vi "Benchmark mupLib_parse_and_eval.vi"(8 "error in (no error)":errorcluster, 10 "Iterations":i32, 11 "Expression":string) -> (0 "error out":errorcluster, 2 "x":dbl[](array[numeric]), 3 "y":dbl[](array[numeric]), 5 "dt average":dbl)   [LabVIEW 2015]
uses:
  mupLib/mupCheckError.vi
  mupLib/mupLibPath.vi
  <vilib>/Utility/error.llb/Error Cluster From Error Code.vi
  mupLib/mupLib.lvlib
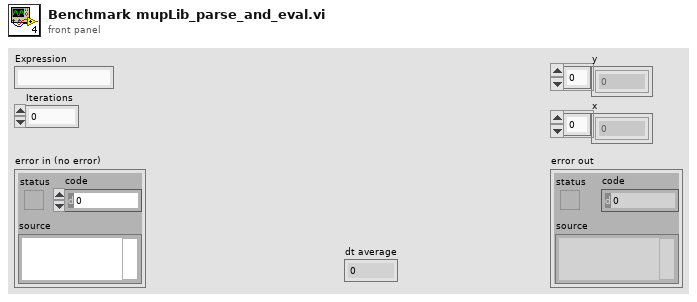
[diagram p1: front panel]
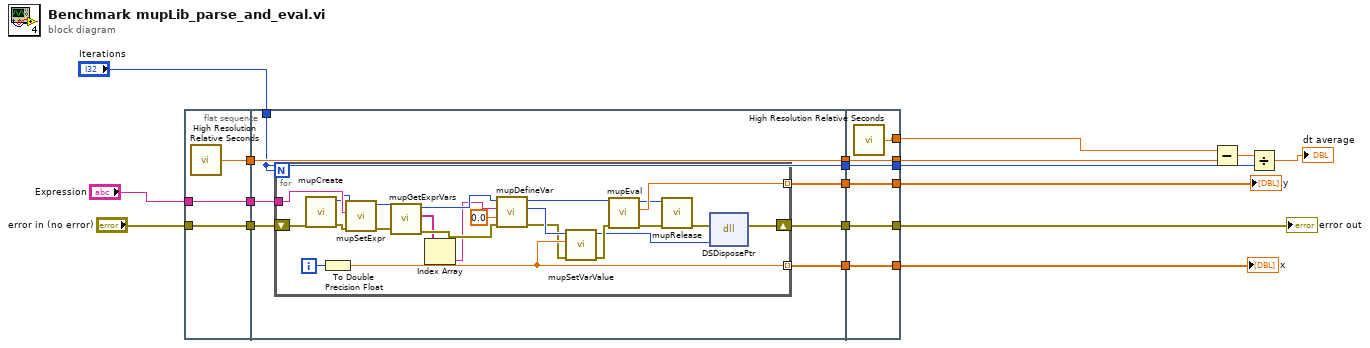
[diagram p0: block diagram]
diagram:
  n1 = flat-sequence {
    tunnel: [w22] -> w17
    tunnel: [w21] -> w12
    tunnel: [w20] -> w1
    tunnel: "error in (no error)" -> [w22]
    tunnel: "Expression" -> [w20]
    tunnel: w17 -> [w29]
    tunnel: [w28] -> w16
    tunnel: [w27] -> w15
    tunnel: [w26] -> w14
    tunnel: [w25] -> w13
    tunnel: w12 -> [w25]
    tunnel: "Iterations" -> [w24]
    tunnel: [w24] -> w6
    tunnel: w1 -> [w23]
    tunnel: w16 -> [w58]
    tunnel: w15 -> [w57]
    tunnel: w14 -> [w56]
    tunnel: w13 -> [w55]
    tunnel: w6 -> [w53]
    tunnel: [w58] -> w2
    tunnel: [w57] -> w19
    tunnel: [w56] -> w18
    tunnel: [w55] -> w10
    tunnel: [w54] -> w11
    tunnel: [w53] -> w7
    frame #0 {
      n2 = call <vilib>:"High Resolution Relative Seconds.vi"() -> ("relative seconds"=w21:dbl)
    }
    frame #1 {
      n3 = for {
        N: w24 -> [_]
        shift-right: [w40] -> w28
        shift-left: w29 -> [w46]
        tunnel: [w49] -> w27 mode=indexing
        tunnel: [w50] -> w26 mode=indexing
        tunnel: w23 -> [w47]
        i -> [w52]
        n4 = call "mupCreate.vi"("error in (no error)"=w46) -> ("error out"=w34:errorcluster, "hParser out"=w35:u64)  [unwired: 9 in]
        n5 = To Double Precision Float(number=w52) -> (double precision float=w50:dbl)
        n6 = call "mupSetExpr.vi"("error in (no error)"=w34, "szExpr"=w47, "muPar in"=w35) -> ("error out"=w32:errorcluster, "muPar out"=w33:u64)  [unwired: 7 in]
        n7 = call "mupGetExprVars.vi"("error in (no error)"=w32, "hParser in"=w33) -> ("error out"=w38:errorcluster, "varNames"=w37:string[], "hParser out"=w39:u64)  [unwired: 5 in, 2 out]
        n8 = Index Array(array=w37) -> (element=w36:string)  [unwired: 1 in]
        n9 = call "mupDefineVar.vi"("error in (no error)"=w38, "initValue"=0.0, "varName"=w36, "hParser in"=w39) -> ("error out"=w30:errorcluster, "varAddr"=w45:u64, "hParser out"=w31:u64)  [unwired: 5 in]
        n10 = call "mupSetVarValue.vi"("error in (no error)"=w30, "varValue"=w50, "varPtr in"=w45) -> ("error out"=w51:errorcluster, "varPtr out"=w42:u64)  [unwired: 7 in]
        n11 = call "mupEval.vi"("error in (no error)"=w51, "hParser in"=w31) -> ("error out"=w43:errorcluster, "result"=w49:dbl, "hParser out"=w44:u64)  [unwired: 7 in]
        n12 = call "mupRelease.vi"("error in (no error)"=w43, "hParser in"=w44) -> ("error out"=w41:errorcluster)  [unwired: 9 in]
        n13 = dll-call lib="LabVIEW" fn="DSDisposePtr"(error in=w41, "ptr"=w42) -> (error out=w40:errorcluster)  [unwired: 4 in, 1 out]
      }
    }
    frame #2 {
      n14 = call <vilib>:"High Resolution Relative Seconds.vi"() -> ("relative seconds"=w54:dbl)
    }
  }
  n15 = Subtract(x=w11, y=w10) -> (x-y=w8:dbl)
  n16 = Divide(x=w8, y=w7) -> (x/y=→"dt average":dbl)
  "y" <- w19
  "x" <- w18
  "error out" <- w2
